vi "Byte_Size_Calculation.vi"() -> ()   [LabVIEW 2014]
uses:
  TSMaster_API/DataBase/Typedef/CAN/TCANSignal.ctl
  TSMaster_API/DataBase/Typedef/LIN/TLINSignal.ctl
  TSMaster_API/DataBase/Typedef/FlexRay/TFlexRaySignal.ctl
panel:
  in  "TDBSignalProperties":T4
  in  "TDBECUProperties":T5
  out "长度":i32
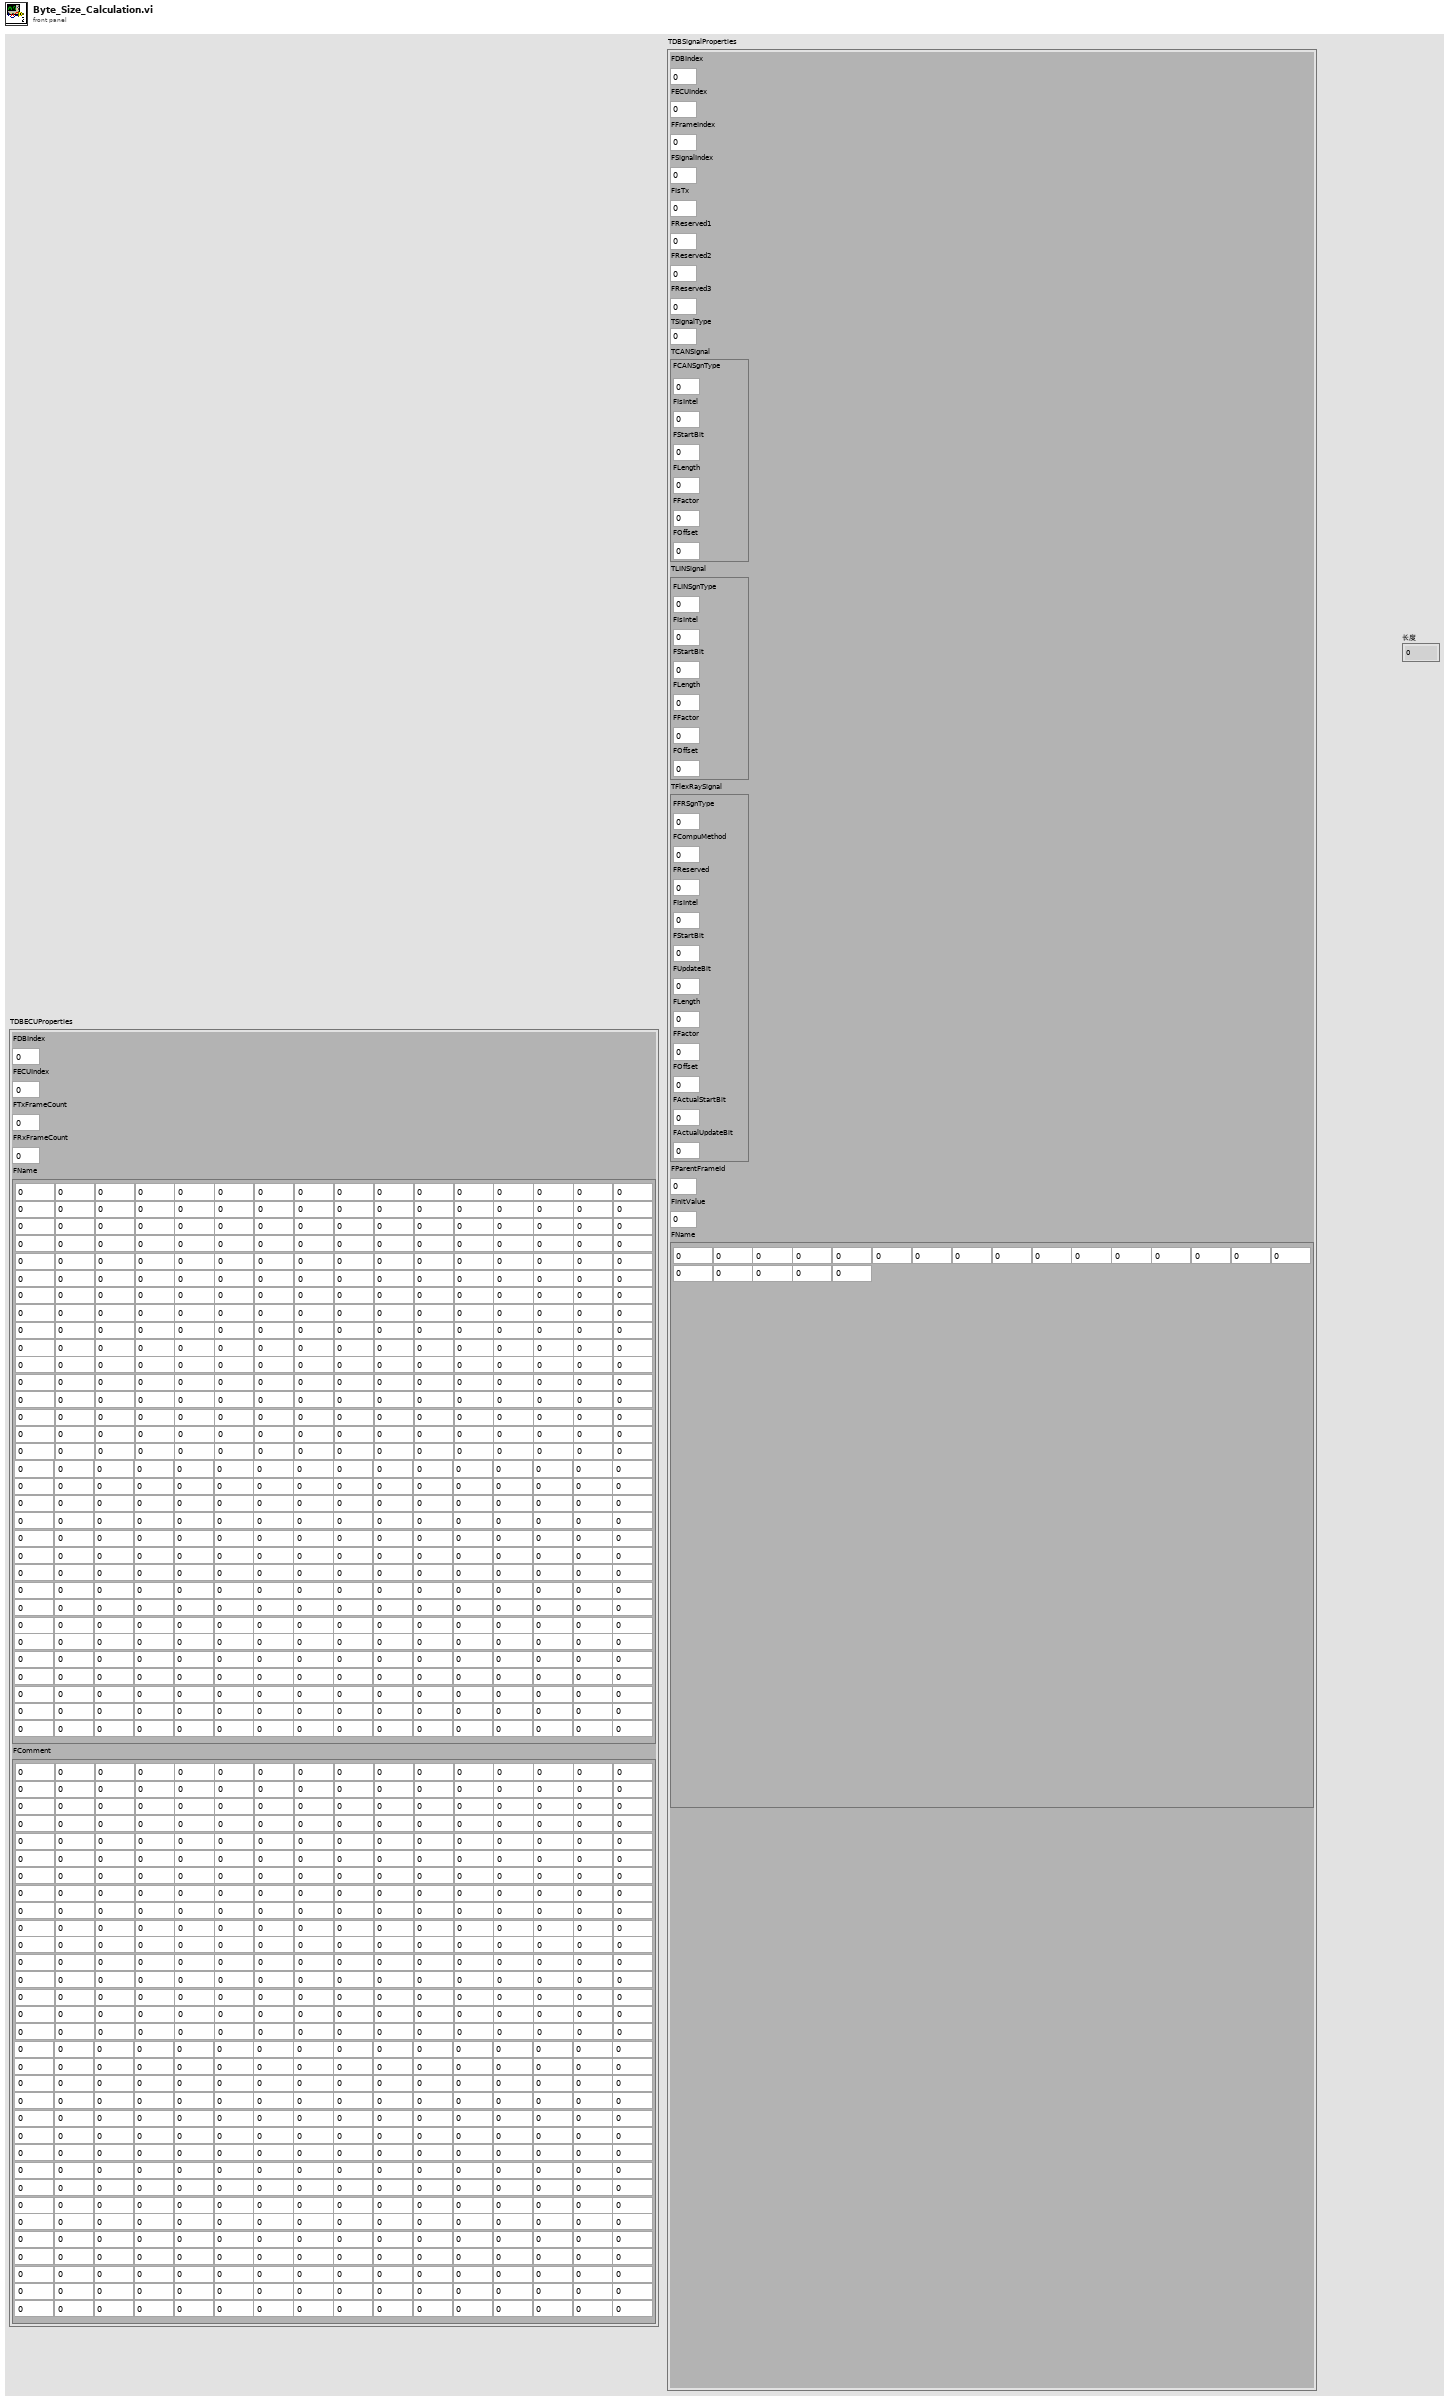
[diagram p1: front panel]
types:
  T1 = typedef "TCANSignal.ctl" = cluster{"FCANSgnType":u8, "FIsIntel":u8, "FStartBit":i32, "FLength":i32, "FFactor":dbl, "FOffset":dbl}
  T2 = typedef "TLINSignal.ctl" = cluster{"FLINSgnType":u8, "FIsIntel":u8, "FStartBit":i32, "FLength":i32, "FFactor":dbl, "FOffset":dbl}
  T3 = typedef "TFlexRaySignal.ctl" = cluster{"FFRSgnType":u8, "FCompuMethod":u8, "FReserved":u8, "FIsIntel":u8, "FStartBit":i32, "FUpdateBit":i32, "FLength":i32, "FFactor":dbl, "FOffset":dbl, "FActualStartBit":i32, "FActualUpdateBit":i32}
  T4 = cluster{"FDBIndex":i32, "FECUIndex":i32, "FFrameIndex":i32, "FSignalIndex":i32, "FIsTx":u8, "FReserved1":u8, "FReserved2":u8, "FReserved3":u8, "TSignalType":i32, "TCANSignal":T1, "TLINSignal":T2, "TFlexRaySignal":T3, "FParentFrameId":i32, "FInitValue":dbl, "FName":cluster{"数值":u8, "数值 9":u8, "数值 17":u8, "数值 25":u8, "数值 33":u8, "数值 41":u8, "数值 49":u8, "数值 57":u8, "数值 65":u8, "数值 73":u8, "数值 81":u8, "数值 89":u8, "数值 97":u8, "数值 105":u8, "数值 98":u8, "数值 99":u8, "数值 2":u8, "数值 10":u8, "数值 18":u8, "数值 26":u8, "数值 34":u8, "数值 42":u8, "数值 50":u8, "数值 58":u8, "数值 66":u8, "数值 74":u8, "数值 82":u8, "数值 90":u8, "数值 100":u8, "数值 106":u8, "数值 101":u8, "数值 102":u8, "数值 3":u8, "数值 11":u8, "数值 19":u8, "数值 27":u8, "数值 35":u8, "数值 43":u8, "数值 51":u8, "数值 59":u8, "数值 67":u8, "数值 75":u8, "数值 83":u8, "数值 91":u8, "数值 103":u8, "数值 107":u8, "数值 104":u8, "数值 108":u8, "数值 4":u8, "数值 12":u8, "数值 20":u8, "数值 28":u8, "数值 36":u8, "数值 44":u8, "数值 52":u8, "数值 60":u8, "数值 68":u8, "数值 76":u8, "数值 84":u8, "数值 92":u8, "数值 109":u8, "数值 110":u8, "数值 111":u8, "数值 112":u8, "数值 5":u8, "数值 13":u8, "数值 21":u8, "数值 29":u8, "数值 37":u8, "数值 45":u8, "数值 53":u8, "数值 61":u8, "数值 69":u8, "数值 77":u8, "数值 85":u8, "数值 93":u8, "数值 113":u8, "数值 114":u8, "数值 115":u8, "数值 116":u8, "数值 6":u8, "数值 14":u8, "数值 22":u8, "数值 30":u8, "数值 38":u8, "数值 46":u8, "数值 54":u8, "数值 62":u8, "数值 70":u8, "数值 78":u8, "数值 86":u8, "数值 94":u8, "数值 117":u8, "数值 118":u8, "数值 119":u8, "数值 120":u8, "数值 7":u8, "数值 15":u8, "数值 23":u8, "数值 31":u8, "数值 39":u8, "数值 47":u8, "数值 55":u8, "数值 63":u8, "数值 71":u8, "数值 79":u8, "数值 87":u8, "数值 95":u8, "数值 121":u8, "数值 122":u8, "数值 123":u8, "数值 124":u8, "数值 8":u8, "数值 16":u8, "数值 24":u8, "数值 32":u8, "数值 40":u8, "数值 48":u8, "数值 56":u8, "数值 64":u8, "数值 72":u8, "数值 80":u8, "数值 88":u8, "数值 96":u8, "数值 125":u8, "数值 126":u8, "数值 127":u8, "数值 128":u8, "数值 129":u8, "数值 130":u8, "数值 131":u8, "数值 132":u8, "数值 133":u8, "数值 134":u8, "数值 135":u8, "数值 136":u8, "数值 137":u8, "数值 138":u8, "数值 139":u8, "数值 140":u8, "数值 141":u8, "数值 142":u8, "数值 143":u8, "数值 144":u8, "数值 145":u8, "数值 146":u8, "数值 147":u8, "数值 148":u8, "数值 149":u8, "数值 150":u8, "数值 151":u8, "数值 152":u8, "数值 153":u8, "数值 154":u8, "数值 155":u8, "数值 156":u8, "数值 157":u8, "数值 158":u8, "数值 159":u8, "数值 160":u8, "数值 161":u8, "数值 162":u8, "数值 163":u8, "数值 164":u8, "数值 165":u8, "数值 166":u8, "数值 167":u8, "数值 168":u8, "数值 169":u8, "数值 170":u8, "数值 171":u8, "数值 172":u8, "数值 173":u8, "数值 174":u8, "数值 175":u8, "数值 176":u8, "数值 177":u8, "数值 178":u8, "数值 179":u8, "数值 180":u8, "数值 181":u8, "数值 182":u8, "数值 183":u8, "数值 184":u8, "数值 185":u8, "数值 186":u8, "数值 187":u8, "数值 188":u8, "数值 189":u8, "数值 190":u8, "数值 191":u8, "数值 192":u8, "数值 193":u8, "数值 194":u8, "数值 195":u8, "数值 196":u8, "数值 197":u8, "数值 198":u8, "数值 199":u8, "数值 200":u8, "数值 201":u8, "数值 202":u8, "数值 203":u8, "数值 204":u8, "数值 205":u8, "数值 206":u8, "数值 207":u8, "数值 208":u8, "数值 209":u8, "数值 210":u8, "数值 211":u8, "数值 212":u8, "数值 213":u8, "数值 214":u8, "数值 215":u8, "数值 216":u8, "数值 217":u8, "数值 218":u8, "数值 219":u8, "数值 220":u8, "数值 221":u8, "数值 222":u8, "数值 223":u8, "数值 224":u8, "数值 225":u8, "数值 226":u8, "数值 227":u8, "数值 228":u8, "数值 229":u8, "数值 230":u8, "数值 231":u8, "数值 232":u8, "数值 233":u8, "数值 234":u8, "数值 235":u8, "数值 236":u8, "数值 237":u8, "数值 238":u8, "数值 239":u8, "数值 240":u8, "数值 241":u8, "数值 242":u8, "数值 243":u8, "数值 244":u8, "数值 245":u8, "数值 246":u8, "数值 247":u8, "数值 248":u8, "数值 249":u8, "数值 250":u8, "数值 251":u8, "数值 252":u8, "数值 253":u8, "数值 254":u8, "数值 255":u8, "数值 256":u8, "数值 257":u8, "数值 258":u8, "数值 259":u8, "数值 260":u8, "数值 261":u8, "数值 262":u8, "数值 263":u8, "数值 264":u8, "数值 265":u8, "数值 266":u8, "数值 267":u8, "数值 268":u8, "数值 269":u8, "数值 270":u8, "数值 271":u8, "数值 272":u8, "数值 273":u8, "数值 274":u8, "数值 275":u8, "数值 276":u8, "数值 277":u8, "数值 278":u8, "数值 279":u8, "数值 280":u8, "数值 281":u8, "数值 282":u8, "数值 283":u8, "数值 284":u8, "数值 285":u8, "数值 286":u8, "数值 287":u8, "数值 288":u8, "数值 289":u8, "数值 290":u8, "数值 291":u8, "数值 292":u8, "数值 293":u8, "数值 294":u8, "数值 295":u8, "数值 296":u8, "数值 297":u8, "数值 298":u8, "数值 299":u8, "数值 300":u8, "数值 301":u8, "数值 302":u8, "数值 303":u8, "数值 304":u8, "数值 305":u8, "数值 306":u8, "数值 307":u8, "数值 308":u8, "数值 309":u8, "数值 310":u8, "数值 311":u8, "数值 312":u8, "数值 313":u8, "数值 314":u8, "数值 315":u8, "数值 316":u8, "数值 317":u8, "数值 318":u8, "数值 319":u8, "数值 320":u8, "数值 321":u8, "数值 322":u8, "数值 323":u8, "数值 324":u8, "数值 325":u8, "数值 326":u8, "数值 327":u8, "数值 328":u8, "数值 329":u8, "数值 330":u8, "数值 331":u8, "数值 332":u8, "数值 333":u8, "数值 334":u8, "数值 335":u8, "数值 336":u8, "数值 337":u8, "数值 338":u8, "数值 339":u8, "数值 340":u8, "数值 341":u8, "数值 342":u8, "数值 343":u8, "数值 344":u8, "数值 345":u8, "数值 346":u8, "数值 347":u8, "数值 348":u8, "数值 349":u8, "数值 350":u8, "数值 351":u8, "数值 352":u8, "数值 353":u8, "数值 354":u8, "数值 355":u8, "数值 356":u8, "数值 357":u8, "数值 358":u8, "数值 359":u8, "数值 360":u8, "数值 361":u8, "数值 362":u8, "数值 363":u8, "数值 364":u8, "数值 365":u8, "数值 366":u8, "数值 367":u8, "数值 368":u8, "数值 369":u8, "数值 370":u8, "数值 371":u8, "数值 372":u8, "数值 373":u8, "数值 374":u8, "数值 375":u8, "数值 376":u8, "数值 377":u8, "数值 378":u8, "数值 379":u8, "数值 380":u8, "数值 381":u8, "数值 382":u8, "数值 383":u8, "数值 384":u8, "数值 385":u8, "数值 386":u8, "数值 387":u8, "数值 388":u8, "数值 389":u8, "数值 390":u8, "数值 391":u8, "数值 392":u8, "数值 393":u8, "数值 394":u8, "数值 395":u8, "数值 396":u8, "数值 397":u8, "数值 398":u8, "数值 399":u8, "数值 400":u8, "数值 401":u8, "数值 402":u8, "数值 403":u8, "数值 404":u8, "数值 405":u8, "数值 406":u8, "数值 407":u8, "数值 408":u8, "数值 409":u8, "数值 410":u8, "数值 411":u8, "数值 412":u8, "数值 413":u8, "数值 414":u8, "数值 415":u8, "数值 416":u8, "数值 417":u8, "数值 418":u8, "数值 419":u8, "数值 420":u8, "数值 421":u8, "数值 422":u8, "数值 423":u8, "数值 424":u8, "数值 425":u8, "数值 426":u8, "数值 427":u8, "数值 428":u8, "数值 429":u8, "数值 430":u8, "数值 431":u8, "数值 432":u8, "数值 433":u8, "数值 434":u8, "数值 435":u8, "数值 436":u8, "数值 437":u8, "数值 438":u8, "数值 439":u8, "数值 440":u8, "数值 441":u8, "数值 442":u8, "数值 443":u8, "数值 444":u8, "数值 445":u8, "数值 446":u8, "数值 447":u8, "数值 448":u8, "数值 449":u8, "数值 450":u8, "数值 451":u8, "数值 452":u8, "数值 453":u8, "数值 454":u8, "数值 455":u8, "数值 456":u8, "数值 457":u8, "数值 458":u8, "数值 459":u8, "数值 460":u8, "数值 461":u8, "数值 462":u8, "数值 463":u8, "数值 464":u8, "数值 465":u8, "数值 466":u8, "数值 467":u8, "数值 468":u8, "数值 469":u8, "数值 470":u8, "数值 471":u8, "数值 472":u8, "数值 473":u8, "数值 474":u8, "数值 475":u8, "数值 476":u8, "数值 477":u8, "数值 478":u8, "数值 479":u8, "数值 480":u8, "数值 481":u8, "数值 482":u8, "数值 483":u8, "数值 484":u8, "数值 485":u8, "数值 486":u8, "数值 487":u8, "数值 488":u8, "数值 489":u8, "数值 490":u8, "数值 491":u8, "数值 492":u8, "数值 493":u8, "数值 494":u8, "数值 495":u8, "数值 496":u8, "数值 497":u8, "数值 498":u8, "数值 499":u8, "数值 500":u8, "数值 501":u8, "数值 502":u8, "数值 503":u8, "数值 504":u8, "数值 505":u8, "数值 506":u8, "数值 507":u8, "数值 508":u8, "数值 509":u8, "数值 510":u8, "数值 511":u8, "数值 512":u8}, "FComment":cluster{"数值":u8, "数值 9":u8, "数值 17":u8, "数值 25":u8, "数值 33":u8, "数值 41":u8, "数值 49":u8, "数值 57":u8, "数值 65":u8, "数值 73":u8, "数值 81":u8, "数值 89":u8, "数值 97":u8, "数值 105":u8, "数值 98":u8, "数值 99":u8, "数值 2":u8, "数值 10":u8, "数值 18":u8, "数值 26":u8, "数值 34":u8, "数值 42":u8, "数值 50":u8, "数值 58":u8, "数值 66":u8, "数值 74":u8, "数值 82":u8, "数值 90":u8, "数值 100":u8, "数值 106":u8, "数值 101":u8, "数值 102":u8, "数值 3":u8, "数值 11":u8, "数值 19":u8, "数值 27":u8, "数值 35":u8, "数值 43":u8, "数值 51":u8, "数值 59":u8, "数值 67":u8, "数值 75":u8, "数值 83":u8, "数值 91":u8, "数值 103":u8, "数值 107":u8, "数值 104":u8, "数值 108":u8, "数值 4":u8, "数值 12":u8, "数值 20":u8, "数值 28":u8, "数值 36":u8, "数值 44":u8, "数值 52":u8, "数值 60":u8, "数值 68":u8, "数值 76":u8, "数值 84":u8, "数值 92":u8, "数值 109":u8, "数值 110":u8, "数值 111":u8, "数值 112":u8, "数值 5":u8, "数值 13":u8, "数值 21":u8, "数值 29":u8, "数值 37":u8, "数值 45":u8, "数值 53":u8, "数值 61":u8, "数值 69":u8, "数值 77":u8, "数值 85":u8, "数值 93":u8, "数值 113":u8, "数值 114":u8, "数值 115":u8, "数值 116":u8, "数值 6":u8, "数值 14":u8, "数值 22":u8, "数值 30":u8, "数值 38":u8, "数值 46":u8, "数值 54":u8, "数值 62":u8, "数值 70":u8, "数值 78":u8, "数值 86":u8, "数值 94":u8, "数值 117":u8, "数值 118":u8, "数值 119":u8, "数值 120":u8, "数值 7":u8, "数值 15":u8, "数值 23":u8, "数值 31":u8, "数值 39":u8, "数值 47":u8, "数值 55":u8, "数值 63":u8, "数值 71":u8, "数值 79":u8, "数值 87":u8, "数值 95":u8, "数值 121":u8, "数值 122":u8, "数值 123":u8, "数值 124":u8, "数值 8":u8, "数值 16":u8, "数值 24":u8, "数值 32":u8, "数值 40":u8, "数值 48":u8, "数值 56":u8, "数值 64":u8, "数值 72":u8, "数值 80":u8, "数值 88":u8, "数值 96":u8, "数值 125":u8, "数值 126":u8, "数值 127":u8, "数值 128":u8, "数值 129":u8, "数值 130":u8, "数值 131":u8, "数值 132":u8, "数值 133":u8, "数值 134":u8, "数值 135":u8, "数值 136":u8, "数值 137":u8, "数值 138":u8, "数值 139":u8, "数值 140":u8, "数值 141":u8, "数值 142":u8, "数值 143":u8, "数值 144":u8, "数值 145":u8, "数值 146":u8, "数值 147":u8, "数值 148":u8, "数值 149":u8, "数值 150":u8, "数值 151":u8, "数值 152":u8, "数值 153":u8, "数值 154":u8, "数值 155":u8, "数值 156":u8, "数值 157":u8, "数值 158":u8, "数值 159":u8, "数值 160":u8, "数值 161":u8, "数值 162":u8, "数值 163":u8, "数值 164":u8, "数值 165":u8, "数值 166":u8, "数值 167":u8, "数值 168":u8, "数值 169":u8, "数值 170":u8, "数值 171":u8, "数值 172":u8, "数值 173":u8, "数值 174":u8, "数值 175":u8, "数值 176":u8, "数值 177":u8, "数值 178":u8, "数值 179":u8, "数值 180":u8, "数值 181":u8, "数值 182":u8, "数值 183":u8, "数值 184":u8, "数值 185":u8, "数值 186":u8, "数值 187":u8, "数值 188":u8, "数值 189":u8, "数值 190":u8, "数值 191":u8, "数值 192":u8, "数值 193":u8, "数值 194":u8, "数值 195":u8, "数值 196":u8, "数值 197":u8, "数值 198":u8, "数值 199":u8, "数值 200":u8, "数值 201":u8, "数值 202":u8, "数值 203":u8, "数值 204":u8, "数值 205":u8, "数值 206":u8, "数值 207":u8, "数值 208":u8, "数值 209":u8, "数值 210":u8, "数值 211":u8, "数值 212":u8, "数值 213":u8, "数值 214":u8, "数值 215":u8, "数值 216":u8, "数值 217":u8, "数值 218":u8, "数值 219":u8, "数值 220":u8, "数值 221":u8, "数值 222":u8, "数值 223":u8, "数值 224":u8, "数值 225":u8, "数值 226":u8, "数值 227":u8, "数值 228":u8, "数值 229":u8, "数值 230":u8, "数值 231":u8, "数值 232":u8, "数值 233":u8, "数值 234":u8, "数值 235":u8, "数值 236":u8, "数值 237":u8, "数值 238":u8, "数值 239":u8, "数值 240":u8, "数值 241":u8, "数值 242":u8, "数值 243":u8, "数值 244":u8, "数值 245":u8, "数值 246":u8, "数值 247":u8, "数值 248":u8, "数值 249":u8, "数值 250":u8, "数值 251":u8, "数值 252":u8, "数值 253":u8, "数值 254":u8, "数值 255":u8, "数值 256":u8, "数值 257":u8, "数值 258":u8, "数值 259":u8, "数值 260":u8, "数值 261":u8, "数值 262":u8, "数值 263":u8, "数值 264":u8, "数值 265":u8, "数值 266":u8, "数值 267":u8, "数值 268":u8, "数值 269":u8, "数值 270":u8, "数值 271":u8, "数值 272":u8, "数值 273":u8, "数值 274":u8, "数值 275":u8, "数值 276":u8, "数值 277":u8, "数值 278":u8, "数值 279":u8, "数值 280":u8, "数值 281":u8, "数值 282":u8, "数值 283":u8, "数值 284":u8, "数值 285":u8, "数值 286":u8, "数值 287":u8, "数值 288":u8, "数值 289":u8, "数值 290":u8, "数值 291":u8, "数值 292":u8, "数值 293":u8, "数值 294":u8, "数值 295":u8, "数值 296":u8, "数值 297":u8, "数值 298":u8, "数值 299":u8, "数值 300":u8, "数值 301":u8, "数值 302":u8, "数值 303":u8, "数值 304":u8, "数值 305":u8, "数值 306":u8, "数值 307":u8, "数值 308":u8, "数值 309":u8, "数值 310":u8, "数值 311":u8, "数值 312":u8, "数值 313":u8, "数值 314":u8, "数值 315":u8, "数值 316":u8, "数值 317":u8, "数值 318":u8, "数值 319":u8, "数值 320":u8, "数值 321":u8, "数值 322":u8, "数值 323":u8, "数值 324":u8, "数值 325":u8, "数值 326":u8, "数值 327":u8, "数值 328":u8, "数值 329":u8, "数值 330":u8, "数值 331":u8, "数值 332":u8, "数值 333":u8, "数值 334":u8, "数值 335":u8, "数值 336":u8, "数值 337":u8, "数值 338":u8, "数值 339":u8, "数值 340":u8, "数值 341":u8, "数值 342":u8, "数值 343":u8, "数值 344":u8, "数值 345":u8, "数值 346":u8, "数值 347":u8, "数值 348":u8, "数值 349":u8, "数值 350":u8, "数值 351":u8, "数值 352":u8, "数值 353":u8, "数值 354":u8, "数值 355":u8, "数值 356":u8, "数值 357":u8, "数值 358":u8, "数值 359":u8, "数值 360":u8, "数值 361":u8, "数值 362":u8, "数值 363":u8, "数值 364":u8, "数值 365":u8, "数值 366":u8, "数值 367":u8, "数值 368":u8, "数值 369":u8, "数值 370":u8, "数值 371":u8, "数值 372":u8, "数值 373":u8, "数值 374":u8, "数值 375":u8, "数值 376":u8, "数值 377":u8, "数值 378":u8, "数值 379":u8, "数值 380":u8, "数值 381":u8, "数值 382":u8, "数值 383":u8, "数值 384":u8, "数值 385":u8, "数值 386":u8, "数值 387":u8, "数值 388":u8, "数值 389":u8, "数值 390":u8, "数值 391":u8, "数值 392":u8, "数值 393":u8, "数值 394":u8, "数值 395":u8, "数值 396":u8, "数值 397":u8, "数值 398":u8, "数值 399":u8, "数值 400":u8, "数值 401":u8, "数值 402":u8, "数值 403":u8, "数值 404":u8, "数值 405":u8, "数值 406":u8, "数值 407":u8, "数值 408":u8, "数值 409":u8, "数值 410":u8, "数值 411":u8, "数值 412":u8, "数值 413":u8, "数值 414":u8, "数值 415":u8, "数值 416":u8, "数值 417":u8, "数值 418":u8, "数值 419":u8, "数值 420":u8, "数值 421":u8, "数值 422":u8, "数值 423":u8, "数值 424":u8, "数值 425":u8, "数值 426":u8, "数值 427":u8, "数值 428":u8, "数值 429":u8, "数值 430":u8, "数值 431":u8, "数值 432":u8, "数值 433":u8, "数值 434":u8, "数值 435":u8, "数值 436":u8, "数值 437":u8, "数值 438":u8, "数值 439":u8, "数值 440":u8, "数值 441":u8, "数值 442":u8, "数值 443":u8, "数值 444":u8, "数值 445":u8, "数值 446":u8, "数值 447":u8, "数值 448":u8, "数值 449":u8, "数值 450":u8, "数值 451":u8, "数值 452":u8, "数值 453":u8, "数值 454":u8, "数值 455":u8, "数值 456":u8, "数值 457":u8, "数值 458":u8, "数值 459":u8, "数值 460":u8, "数值 461":u8, "数值 462":u8, "数值 463":u8, "数值 464":u8, "数值 465":u8, "数值 466":u8, "数值 467":u8, "数值 468":u8, "数值 469":u8, "数值 470":u8, "数值 471":u8, "数值 472":u8, "数值 473":u8, "数值 474":u8, "数值 475":u8, "数值 476":u8, "数值 477":u8, "数值 478":u8, "数值 479":u8, "数值 480":u8, "数值 481":u8, "数值 482":u8, "数值 483":u8, "数值 484":u8, "数值 485":u8, "数值 486":u8, "数值 487":u8, "数值 488":u8, "数值 489":u8, "数值 490":u8, "数值 491":u8, "数值 492":u8, "数值 493":u8, "数值 494":u8, "数值 495":u8, "数值 496":u8, "数值 497":u8, "数值 498":u8, "数值 499":u8, "数值 500":u8, "数值 501":u8, "数值 502":u8, "数值 503":u8, "数值 504":u8, "数值 505":u8, "数值 506":u8, "数值 507":u8, "数值 508":u8, "数值 509":u8, "数值 510":u8, "数值 511":u8, "数值 512":u8}}
  T5 = cluster{"FDBIndex":i32, "FECUIndex":i32, "FTxFrameCount":i32, "FRxFrameCount":i32, "FName":cluster{"数值":u8, "数值 9":u8, "数值 17":u8, "数值 25":u8, "数值 33":u8, "数值 41":u8, "数值 49":u8, "数值 57":u8, "数值 65":u8, "数值 73":u8, "数值 81":u8, "数值 89":u8, "数值 97":u8, "数值 105":u8, "数值 98":u8, "数值 99":u8, "数值 2":u8, "数值 10":u8, "数值 18":u8, "数值 26":u8, "数值 34":u8, "数值 42":u8, "数值 50":u8, "数值 58":u8, "数值 66":u8, "数值 74":u8, "数值 82":u8, "数值 90":u8, "数值 100":u8, "数值 106":u8, "数值 101":u8, "数值 102":u8, "数值 3":u8, "数值 11":u8, "数值 19":u8, "数值 27":u8, "数值 35":u8, "数值 43":u8, "数值 51":u8, "数值 59":u8, "数值 67":u8, "数值 75":u8, "数值 83":u8, "数值 91":u8, "数值 103":u8, "数值 107":u8, "数值 104":u8, "数值 108":u8, "数值 4":u8, "数值 12":u8, "数值 20":u8, "数值 28":u8, "数值 36":u8, "数值 44":u8, "数值 52":u8, "数值 60":u8, "数值 68":u8, "数值 76":u8, "数值 84":u8, "数值 92":u8, "数值 109":u8, "数值 110":u8, "数值 111":u8, "数值 112":u8, "数值 5":u8, "数值 13":u8, "数值 21":u8, "数值 29":u8, "数值 37":u8, "数值 45":u8, "数值 53":u8, "数值 61":u8, "数值 69":u8, "数值 77":u8, "数值 85":u8, "数值 93":u8, "数值 113":u8, "数值 114":u8, "数值 115":u8, "数值 116":u8, "数值 6":u8, "数值 14":u8, "数值 22":u8, "数值 30":u8, "数值 38":u8, "数值 46":u8, "数值 54":u8, "数值 62":u8, "数值 70":u8, "数值 78":u8, "数值 86":u8, "数值 94":u8, "数值 117":u8, "数值 118":u8, "数值 119":u8, "数值 120":u8, "数值 7":u8, "数值 15":u8, "数值 23":u8, "数值 31":u8, "数值 39":u8, "数值 47":u8, "数值 55":u8, "数值 63":u8, "数值 71":u8, "数值 79":u8, "数值 87":u8, "数值 95":u8, "数值 121":u8, "数值 122":u8, "数值 123":u8, "数值 124":u8, "数值 8":u8, "数值 16":u8, "数值 24":u8, "数值 32":u8, "数值 40":u8, "数值 48":u8, "数值 56":u8, "数值 64":u8, "数值 72":u8, "数值 80":u8, "数值 88":u8, "数值 96":u8, "数值 125":u8, "数值 126":u8, "数值 127":u8, "数值 128":u8, "数值 129":u8, "数值 130":u8, "数值 131":u8, "数值 132":u8, "数值 133":u8, "数值 134":u8, "数值 135":u8, "数值 136":u8, "数值 137":u8, "数值 138":u8, "数值 139":u8, "数值 140":u8, "数值 141":u8, "数值 142":u8, "数值 143":u8, "数值 144":u8, "数值 145":u8, "数值 146":u8, "数值 147":u8, "数值 148":u8, "数值 149":u8, "数值 150":u8, "数值 151":u8, "数值 152":u8, "数值 153":u8, "数值 154":u8, "数值 155":u8, "数值 156":u8, "数值 157":u8, "数值 158":u8, "数值 159":u8, "数值 160":u8, "数值 161":u8, "数值 162":u8, "数值 163":u8, "数值 164":u8, "数值 165":u8, "数值 166":u8, "数值 167":u8, "数值 168":u8, "数值 169":u8, "数值 170":u8, "数值 171":u8, "数值 172":u8, "数值 173":u8, "数值 174":u8, "数值 175":u8, "数值 176":u8, "数值 177":u8, "数值 178":u8, "数值 179":u8, "数值 180":u8, "数值 181":u8, "数值 182":u8, "数值 183":u8, "数值 184":u8, "数值 185":u8, "数值 186":u8, "数值 187":u8, "数值 188":u8, "数值 189":u8, "数值 190":u8, "数值 191":u8, "数值 192":u8, "数值 193":u8, "数值 194":u8, "数值 195":u8, "数值 196":u8, "数值 197":u8, "数值 198":u8, "数值 199":u8, "数值 200":u8, "数值 201":u8, "数值 202":u8, "数值 203":u8, "数值 204":u8, "数值 205":u8, "数值 206":u8, "数值 207":u8, "数值 208":u8, "数值 209":u8, "数值 210":u8, "数值 211":u8, "数值 212":u8, "数值 213":u8, "数值 214":u8, "数值 215":u8, "数值 216":u8, "数值 217":u8, "数值 218":u8, "数值 219":u8, "数值 220":u8, "数值 221":u8, "数值 222":u8, "数值 223":u8, "数值 224":u8, "数值 225":u8, "数值 226":u8, "数值 227":u8, "数值 228":u8, "数值 229":u8, "数值 230":u8, "数值 231":u8, "数值 232":u8, "数值 233":u8, "数值 234":u8, "数值 235":u8, "数值 236":u8, "数值 237":u8, "数值 238":u8, "数值 239":u8, "数值 240":u8, "数值 241":u8, "数值 242":u8, "数值 243":u8, "数值 244":u8, "数值 245":u8, "数值 246":u8, "数值 247":u8, "数值 248":u8, "数值 249":u8, "数值 250":u8, "数值 251":u8, "数值 252":u8, "数值 253":u8, "数值 254":u8, "数值 255":u8, "数值 256":u8, "数值 257":u8, "数值 258":u8, "数值 259":u8, "数值 260":u8, "数值 261":u8, "数值 262":u8, "数值 263":u8, "数值 264":u8, "数值 265":u8, "数值 266":u8, "数值 267":u8, "数值 268":u8, "数值 269":u8, "数值 270":u8, "数值 271":u8, "数值 272":u8, "数值 273":u8, "数值 274":u8, "数值 275":u8, "数值 276":u8, "数值 277":u8, "数值 278":u8, "数值 279":u8, "数值 280":u8, "数值 281":u8, "数值 282":u8, "数值 283":u8, "数值 284":u8, "数值 285":u8, "数值 286":u8, "数值 287":u8, "数值 288":u8, "数值 289":u8, "数值 290":u8, "数值 291":u8, "数值 292":u8, "数值 293":u8, "数值 294":u8, "数值 295":u8, "数值 296":u8, "数值 297":u8, "数值 298":u8, "数值 299":u8, "数值 300":u8, "数值 301":u8, "数值 302":u8, "数值 303":u8, "数值 304":u8, "数值 305":u8, "数值 306":u8, "数值 307":u8, "数值 308":u8, "数值 309":u8, "数值 310":u8, "数值 311":u8, "数值 312":u8, "数值 313":u8, "数值 314":u8, "数值 315":u8, "数值 316":u8, "数值 317":u8, "数值 318":u8, "数值 319":u8, "数值 320":u8, "数值 321":u8, "数值 322":u8, "数值 323":u8, "数值 324":u8, "数值 325":u8, "数值 326":u8, "数值 327":u8, "数值 328":u8, "数值 329":u8, "数值 330":u8, "数值 331":u8, "数值 332":u8, "数值 333":u8, "数值 334":u8, "数值 335":u8, "数值 336":u8, "数值 337":u8, "数值 338":u8, "数值 339":u8, "数值 340":u8, "数值 341":u8, "数值 342":u8, "数值 343":u8, "数值 344":u8, "数值 345":u8, "数值 346":u8, "数值 347":u8, "数值 348":u8, "数值 349":u8, "数值 350":u8, "数值 351":u8, "数值 352":u8, "数值 353":u8, "数值 354":u8, "数值 355":u8, "数值 356":u8, "数值 357":u8, "数值 358":u8, "数值 359":u8, "数值 360":u8, "数值 361":u8, "数值 362":u8, "数值 363":u8, "数值 364":u8, "数值 365":u8, "数值 366":u8, "数值 367":u8, "数值 368":u8, "数值 369":u8, "数值 370":u8, "数值 371":u8, "数值 372":u8, "数值 373":u8, "数值 374":u8, "数值 375":u8, "数值 376":u8, "数值 377":u8, "数值 378":u8, "数值 379":u8, "数值 380":u8, "数值 381":u8, "数值 382":u8, "数值 383":u8, "数值 384":u8, "数值 385":u8, "数值 386":u8, "数值 387":u8, "数值 388":u8, "数值 389":u8, "数值 390":u8, "数值 391":u8, "数值 392":u8, "数值 393":u8, "数值 394":u8, "数值 395":u8, "数值 396":u8, "数值 397":u8, "数值 398":u8, "数值 399":u8, "数值 400":u8, "数值 401":u8, "数值 402":u8, "数值 403":u8, "数值 404":u8, "数值 405":u8, "数值 406":u8, "数值 407":u8, "数值 408":u8, "数值 409":u8, "数值 410":u8, "数值 411":u8, "数值 412":u8, "数值 413":u8, "数值 414":u8, "数值 415":u8, "数值 416":u8, "数值 417":u8, "数值 418":u8, "数值 419":u8, "数值 420":u8, "数值 421":u8, "数值 422":u8, "数值 423":u8, "数值 424":u8, "数值 425":u8, "数值 426":u8, "数值 427":u8, "数值 428":u8, "数值 429":u8, "数值 430":u8, "数值 431":u8, "数值 432":u8, "数值 433":u8, "数值 434":u8, "数值 435":u8, "数值 436":u8, "数值 437":u8, "数值 438":u8, "数值 439":u8, "数值 440":u8, "数值 441":u8, "数值 442":u8, "数值 443":u8, "数值 444":u8, "数值 445":u8, "数值 446":u8, "数值 447":u8, "数值 448":u8, "数值 449":u8, "数值 450":u8, "数值 451":u8, "数值 452":u8, "数值 453":u8, "数值 454":u8, "数值 455":u8, "数值 456":u8, "数值 457":u8, "数值 458":u8, "数值 459":u8, "数值 460":u8, "数值 461":u8, "数值 462":u8, "数值 463":u8, "数值 464":u8, "数值 465":u8, "数值 466":u8, "数值 467":u8, "数值 468":u8, "数值 469":u8, "数值 470":u8, "数值 471":u8, "数值 472":u8, "数值 473":u8, "数值 474":u8, "数值 475":u8, "数值 476":u8, "数值 477":u8, "数值 478":u8, "数值 479":u8, "数值 480":u8, "数值 481":u8, "数值 482":u8, "数值 483":u8, "数值 484":u8, "数值 485":u8, "数值 486":u8, "数值 487":u8, "数值 488":u8, "数值 489":u8, "数值 490":u8, "数值 491":u8, "数值 492":u8, "数值 493":u8, "数值 494":u8, "数值 495":u8, "数值 496":u8, "数值 497":u8, "数值 498":u8, "数值 499":u8, "数值 500":u8, "数值 501":u8, "数值 502":u8, "数值 503":u8, "数值 504":u8, "数值 505":u8, "数值 506":u8, "数值 507":u8, "数值 508":u8, "数值 509":u8, "数值 510":u8, "数值 511":u8, "数值 512":u8}, "FComment":cluster{"数值":u8, "数值 9":u8, "数值 17":u8, "数值 25":u8, "数值 33":u8, "数值 41":u8, "数值 49":u8, "数值 57":u8, "数值 65":u8, "数值 73":u8, "数值 81":u8, "数值 89":u8, "数值 97":u8, "数值 105":u8, "数值 98":u8, "数值 99":u8, "数值 2":u8, "数值 10":u8, "数值 18":u8, "数值 26":u8, "数值 34":u8, "数值 42":u8, "数值 50":u8, "数值 58":u8, "数值 66":u8, "数值 74":u8, "数值 82":u8, "数值 90":u8, "数值 100":u8, "数值 106":u8, "数值 101":u8, "数值 102":u8, "数值 3":u8, "数值 11":u8, "数值 19":u8, "数值 27":u8, "数值 35":u8, "数值 43":u8, "数值 51":u8, "数值 59":u8, "数值 67":u8, "数值 75":u8, "数值 83":u8, "数值 91":u8, "数值 103":u8, "数值 107":u8, "数值 104":u8, "数值 108":u8, "数值 4":u8, "数值 12":u8, "数值 20":u8, "数值 28":u8, "数值 36":u8, "数值 44":u8, "数值 52":u8, "数值 60":u8, "数值 68":u8, "数值 76":u8, "数值 84":u8, "数值 92":u8, "数值 109":u8, "数值 110":u8, "数值 111":u8, "数值 112":u8, "数值 5":u8, "数值 13":u8, "数值 21":u8, "数值 29":u8, "数值 37":u8, "数值 45":u8, "数值 53":u8, "数值 61":u8, "数值 69":u8, "数值 77":u8, "数值 85":u8, "数值 93":u8, "数值 113":u8, "数值 114":u8, "数值 115":u8, "数值 116":u8, "数值 6":u8, "数值 14":u8, "数值 22":u8, "数值 30":u8, "数值 38":u8, "数值 46":u8, "数值 54":u8, "数值 62":u8, "数值 70":u8, "数值 78":u8, "数值 86":u8, "数值 94":u8, "数值 117":u8, "数值 118":u8, "数值 119":u8, "数值 120":u8, "数值 7":u8, "数值 15":u8, "数值 23":u8, "数值 31":u8, "数值 39":u8, "数值 47":u8, "数值 55":u8, "数值 63":u8, "数值 71":u8, "数值 79":u8, "数值 87":u8, "数值 95":u8, "数值 121":u8, "数值 122":u8, "数值 123":u8, "数值 124":u8, "数值 8":u8, "数值 16":u8, "数值 24":u8, "数值 32":u8, "数值 40":u8, "数值 48":u8, "数值 56":u8, "数值 64":u8, "数值 72":u8, "数值 80":u8, "数值 88":u8, "数值 96":u8, "数值 125":u8, "数值 126":u8, "数值 127":u8, "数值 128":u8, "数值 129":u8, "数值 130":u8, "数值 131":u8, "数值 132":u8, "数值 133":u8, "数值 134":u8, "数值 135":u8, "数值 136":u8, "数值 137":u8, "数值 138":u8, "数值 139":u8, "数值 140":u8, "数值 141":u8, "数值 142":u8, "数值 143":u8, "数值 144":u8, "数值 145":u8, "数值 146":u8, "数值 147":u8, "数值 148":u8, "数值 149":u8, "数值 150":u8, "数值 151":u8, "数值 152":u8, "数值 153":u8, "数值 154":u8, "数值 155":u8, "数值 156":u8, "数值 157":u8, "数值 158":u8, "数值 159":u8, "数值 160":u8, "数值 161":u8, "数值 162":u8, "数值 163":u8, "数值 164":u8, "数值 165":u8, "数值 166":u8, "数值 167":u8, "数值 168":u8, "数值 169":u8, "数值 170":u8, "数值 171":u8, "数值 172":u8, "数值 173":u8, "数值 174":u8, "数值 175":u8, "数值 176":u8, "数值 177":u8, "数值 178":u8, "数值 179":u8, "数值 180":u8, "数值 181":u8, "数值 182":u8, "数值 183":u8, "数值 184":u8, "数值 185":u8, "数值 186":u8, "数值 187":u8, "数值 188":u8, "数值 189":u8, "数值 190":u8, "数值 191":u8, "数值 192":u8, "数值 193":u8, "数值 194":u8, "数值 195":u8, "数值 196":u8, "数值 197":u8, "数值 198":u8, "数值 199":u8, "数值 200":u8, "数值 201":u8, "数值 202":u8, "数值 203":u8, "数值 204":u8, "数值 205":u8, "数值 206":u8, "数值 207":u8, "数值 208":u8, "数值 209":u8, "数值 210":u8, "数值 211":u8, "数值 212":u8, "数值 213":u8, "数值 214":u8, "数值 215":u8, "数值 216":u8, "数值 217":u8, "数值 218":u8, "数值 219":u8, "数值 220":u8, "数值 221":u8, "数值 222":u8, "数值 223":u8, "数值 224":u8, "数值 225":u8, "数值 226":u8, "数值 227":u8, "数值 228":u8, "数值 229":u8, "数值 230":u8, "数值 231":u8, "数值 232":u8, "数值 233":u8, "数值 234":u8, "数值 235":u8, "数值 236":u8, "数值 237":u8, "数值 238":u8, "数值 239":u8, "数值 240":u8, "数值 241":u8, "数值 242":u8, "数值 243":u8, "数值 244":u8, "数值 245":u8, "数值 246":u8, "数值 247":u8, "数值 248":u8, "数值 249":u8, "数值 250":u8, "数值 251":u8, "数值 252":u8, "数值 253":u8, "数值 254":u8, "数值 255":u8, "数值 256":u8, "数值 257":u8, "数值 258":u8, "数值 259":u8, "数值 260":u8, "数值 261":u8, "数值 262":u8, "数值 263":u8, "数值 264":u8, "数值 265":u8, "数值 266":u8, "数值 267":u8, "数值 268":u8, "数值 269":u8, "数值 270":u8, "数值 271":u8, "数值 272":u8, "数值 273":u8, "数值 274":u8, "数值 275":u8, "数值 276":u8, "数值 277":u8, "数值 278":u8, "数值 279":u8, "数值 280":u8, "数值 281":u8, "数值 282":u8, "数值 283":u8, "数值 284":u8, "数值 285":u8, "数值 286":u8, "数值 287":u8, "数值 288":u8, "数值 289":u8, "数值 290":u8, "数值 291":u8, "数值 292":u8, "数值 293":u8, "数值 294":u8, "数值 295":u8, "数值 296":u8, "数值 297":u8, "数值 298":u8, "数值 299":u8, "数值 300":u8, "数值 301":u8, "数值 302":u8, "数值 303":u8, "数值 304":u8, "数值 305":u8, "数值 306":u8, "数值 307":u8, "数值 308":u8, "数值 309":u8, "数值 310":u8, "数值 311":u8, "数值 312":u8, "数值 313":u8, "数值 314":u8, "数值 315":u8, "数值 316":u8, "数值 317":u8, "数值 318":u8, "数值 319":u8, "数值 320":u8, "数值 321":u8, "数值 322":u8, "数值 323":u8, "数值 324":u8, "数值 325":u8, "数值 326":u8, "数值 327":u8, "数值 328":u8, "数值 329":u8, "数值 330":u8, "数值 331":u8, "数值 332":u8, "数值 333":u8, "数值 334":u8, "数值 335":u8, "数值 336":u8, "数值 337":u8, "数值 338":u8, "数值 339":u8, "数值 340":u8, "数值 341":u8, "数值 342":u8, "数值 343":u8, "数值 344":u8, "数值 345":u8, "数值 346":u8, "数值 347":u8, "数值 348":u8, "数值 349":u8, "数值 350":u8, "数值 351":u8, "数值 352":u8, "数值 353":u8, "数值 354":u8, "数值 355":u8, "数值 356":u8, "数值 357":u8, "数值 358":u8, "数值 359":u8, "数值 360":u8, "数值 361":u8, "数值 362":u8, "数值 363":u8, "数值 364":u8, "数值 365":u8, "数值 366":u8, "数值 367":u8, "数值 368":u8, "数值 369":u8, "数值 370":u8, "数值 371":u8, "数值 372":u8, "数值 373":u8, "数值 374":u8, "数值 375":u8, "数值 376":u8, "数值 377":u8, "数值 378":u8, "数值 379":u8, "数值 380":u8, "数值 381":u8, "数值 382":u8, "数值 383":u8, "数值 384":u8, "数值 385":u8, "数值 386":u8, "数值 387":u8, "数值 388":u8, "数值 389":u8, "数值 390":u8, "数值 391":u8, "数值 392":u8, "数值 393":u8, "数值 394":u8, "数值 395":u8, "数值 396":u8, "数值 397":u8, "数值 398":u8, "数值 399":u8, "数值 400":u8, "数值 401":u8, "数值 402":u8, "数值 403":u8, "数值 404":u8, "数值 405":u8, "数值 406":u8, "数值 407":u8, "数值 408":u8, "数值 409":u8, "数值 410":u8, "数值 411":u8, "数值 412":u8, "数值 413":u8, "数值 414":u8, "数值 415":u8, "数值 416":u8, "数值 417":u8, "数值 418":u8, "数值 419":u8, "数值 420":u8, "数值 421":u8, "数值 422":u8, "数值 423":u8, "数值 424":u8, "数值 425":u8, "数值 426":u8, "数值 427":u8, "数值 428":u8, "数值 429":u8, "数值 430":u8, "数值 431":u8, "数值 432":u8, "数值 433":u8, "数值 434":u8, "数值 435":u8, "数值 436":u8, "数值 437":u8, "数值 438":u8, "数值 439":u8, "数值 440":u8, "数值 441":u8, "数值 442":u8, "数值 443":u8, "数值 444":u8, "数值 445":u8, "数值 446":u8, "数值 447":u8, "数值 448":u8, "数值 449":u8, "数值 450":u8, "数值 451":u8, "数值 452":u8, "数值 453":u8, "数值 454":u8, "数值 455":u8, "数值 456":u8, "数值 457":u8, "数值 458":u8, "数值 459":u8, "数值 460":u8, "数值 461":u8, "数值 462":u8, "数值 463":u8, "数值 464":u8, "数值 465":u8, "数值 466":u8, "数值 467":u8, "数值 468":u8, "数值 469":u8, "数值 470":u8, "数值 471":u8, "数值 472":u8, "数值 473":u8, "数值 474":u8, "数值 475":u8, "数值 476":u8, "数值 477":u8, "数值 478":u8, "数值 479":u8, "数值 480":u8, "数值 481":u8, "数值 482":u8, "数值 483":u8, "数值 484":u8, "数值 485":u8, "数值 486":u8, "数值 487":u8, "数值 488":u8, "数值 489":u8, "数值 490":u8, "数值 491":u8, "数值 492":u8, "数值 493":u8, "数值 494":u8, "数值 495":u8, "数值 496":u8, "数值 497":u8, "数值 498":u8, "数值 499":u8, "数值 500":u8, "数值 501":u8, "数值 502":u8, "数值 503":u8, "数值 504":u8, "数值 505":u8, "数值 506":u8, "数值 507":u8, "数值 508":u8, "数值 509":u8, "数值 510":u8, "数值 511":u8, "数值 512":u8}}
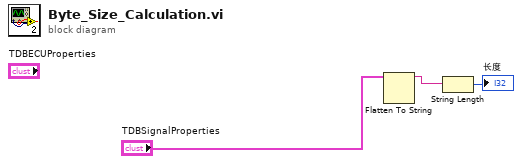
[diagram p0: block diagram]
diagram:
  n1 = Flatten To String(anything="TDBSignalProperties") -> (data string=w3:string)  [unwired: 3 in, 2 out]
  n2 = String Length(string=w3) -> (length=→"长度":i32)
